vi "AsyncBluetoothCallback.vi"(4 "Queue":refnum<queue>, 5 "Event Data":cluster{"_msg":string}, 6 "Control Ref":refnum<k24>, 7 "Event Common Data":T1) -> ()   [LabVIEW 2013]
uses:
  C:/Users/Simon/SkyDrive/LabView/2013/DM2020/bin/medimatic_bt_receiver.dll
  bin/medimatic_bt_receiver.dll
  Controls/Enum User Events.ctl
  main.lvlib
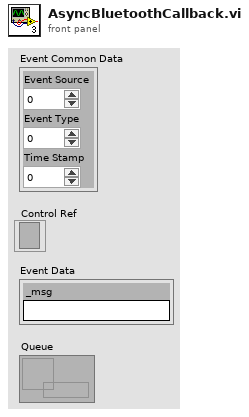
[diagram p1: front panel]
types:
  T1 = cluster{"Event Source":i32, "Event Type":u32, "Time Stamp":u32}
  T2 = typedef "main.lvlib/Enum User Events.ctl" = enum16{"User Event", "Init"}
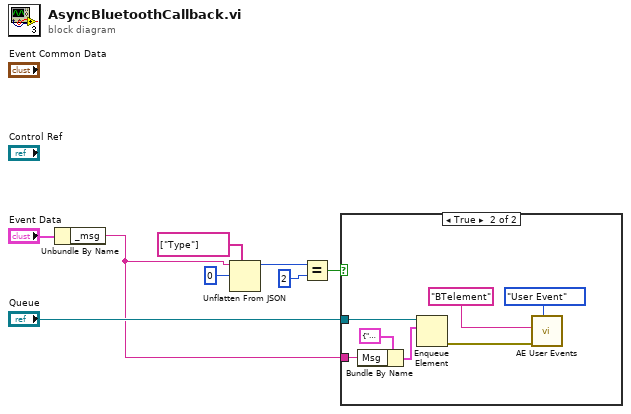
[diagram p0: block diagram]
diagram:
  n1 = Unbundle By Name("Event Data") -> ("_msg"=w4:string)
  n2 = Unflatten From JSON(path=string[] ["Type"], JSON string=w4, type and defaults=0) -> (value=w3:i32)  [unwired: 4 in, 1 out]
  n3 = Equal?(x=w3, y=2) -> (x = y?=w2:bool)
  n4 = case shown="True" w2 {
    tunnel: "Queue" -> [_ w15]
    tunnel: w4 -> [_ w12]
    frame False {
    }
    frame True {
      n5 = Bundle By Name(cluster=cluster{"Cmd":string, "Msg":string} {"Cmd"="BTelement", "Msg"=""}, "Msg"=w12) -> (w13:cluster{"Cmd":string, "Msg":string})
      n6 = Enqueue Element(queue=w15, element=w13) -> (error out=w9:errorcluster)  [unwired: 2 in, 2 out]
      n7 = call "AE User Events.vi"("Action"=Enum_User_Events."User Event", "error in (no error)"=w9, "User Event"="BTelement") -> ()  [unwired: 7 in, 2 out]
    }
  }
